vi "Handle Last Ack Core.vi"(4 "error in":errorcluster, 6 "Last Ack":refnum<class "Last Ack.lvclass">, 7 "MSS Target Actor in":refnum<class "MSS Target Actor.lvclass">) -> (0 "error out":errorcluster, 3 "MSS Target Actor out":refnum<class "MSS Target Actor.lvclass">)   [LabVIEW 2024, in "MSS Target Actor.lvlib" / "MSS Target Actor.lvclass"]
doc: "(<B>Filename</B>: Actor Framework.lvlib:Actor.lvclass:Handle Last Ack Core.vi)\n\nDefines how the caller actor responds to the Last Ack message from a nested actor. The Last Ack message is the final message a nested actor sends to its caller before it shuts down. The message contains information about the final state of the nested actor.\n\nBy default, this method does nothing except return any error the nested actor sent. A descendant class may override this method to define behavior."
uses:
  MSS Target Actor.lvclass
  <vilib>/ActorFramework/LastAck/Last Ack.lvclass
  MSS Target Actor.lvclass/MSS Target Actor.ctl
  <vilib>/ActorFramework/LastAck/Last Ack.lvclass/Last Ack.ctl
  <vilib>/ActorFramework/Actor/Actor.lvclass
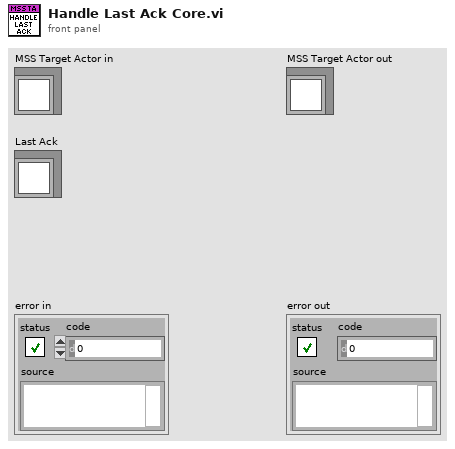
[diagram p1: front panel]
types:
  T1 = map{string, refnum<class "Message Enqueuer.lvclass">}
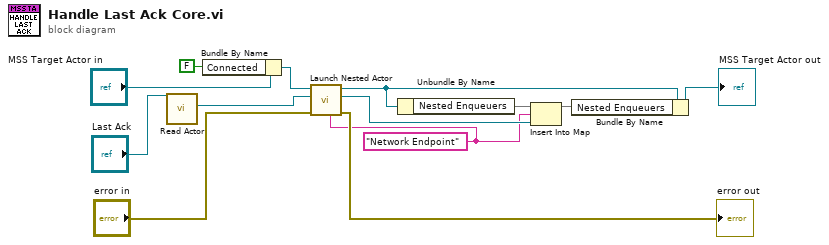
[diagram p0: block diagram]
diagram:
  w4 = "Network Endpoint" ("key")
  n1 = call <vilib>:"Read Actor.vi"("Last Ack"="Last Ack") -> ("Actor"=w3:refnum<class "Actor.lvclass">)  [unwired: 10 in]
  n2 = Bundle By Name(cluster="MSS Target Actor in", "Connected"=FALSE) -> (w2:refnum<class "MSS Target Actor.lvclass">)
  n3 = call <vilib>:"Launch Nested Actor.vi"("Debug Alias"=w4, "error in (no error)"="error in", "Nested Actor"=w3, "Caller Actor in"=w2) -> ("error out"=→"error out":errorcluster, "Nested Actor's Enqueuer"=w6:refnum<class "Message Enqueuer.lvclass">, "Caller Actor out"=w8:refnum<class "MSS Target Actor.lvclass">)  [unwired: 5 in]
  n4 = Unbundle By Name(w8) -> ("Nested Enqueuers"=w7:T1)
  n5 = Insert Into Map(map in=w7, key=w4, value=w6) -> (map out=w5:T1)  [unwired: 2 out]
  n6 = Bundle By Name(cluster=w8, "Nested Enqueuers"=w5) -> (→"MSS Target Actor out":refnum<class "MSS Target Actor.lvclass">)
